vi "checkout.vi"(6 "destroy queue?":bool, 7 "locked by?":string, 8 "error in (no error)":errorcluster) -> (0 "error out":errorcluster, 3 "GenericExperimentController out":refnum<class "GenericExperimentController.lvclass">)   [LabVIEW 2010, in "GenericExperimentController.lvclass"]
uses:
  GenericExperimentController.lvclass
  class_data.vi
  common/classes/GenericComponent/GenericComponent/GenericComponent.lvclass
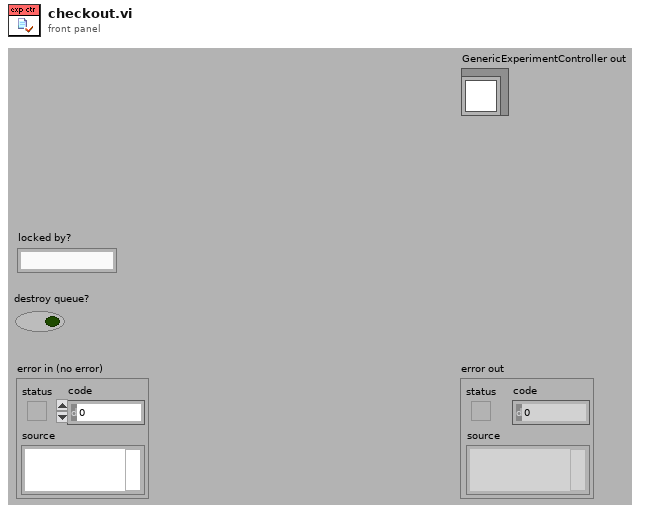
[diagram p1: front panel]
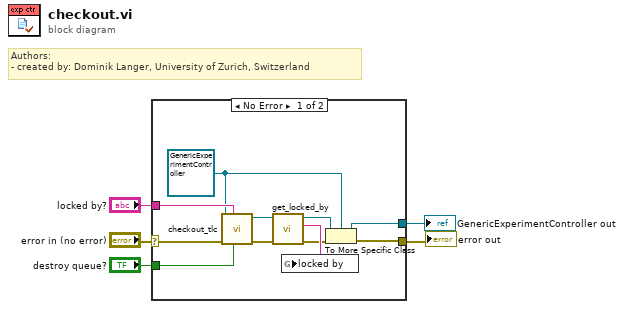
[diagram p0: block diagram]
diagram:
  # "Authors:  \n- created by: Dominik Langer, University of Zurich, Switzerland"
  n1 = case shown="No Error" "error in (no error)" {
    selector: "error in (no error)" -> [w7 w17]
    tunnel: [w15 w17] -> w4
    tunnel: "locked by?" -> [w16 _]
    tunnel: [w14 _] -> w1
    tunnel: "destroy queue?" -> [w8 _]
    frame No Error {
      w6 = refnum<class "GenericExperimentController.lvclass"> refnum ("GenericExperimentController.lvclass")
      n2 = call-dynamic "checkout_tlc.vi"("destroy queue?"=w8, "locked by?"=w16, "error in (no error)"=w7, "GenericToplevelComponent in"=w6) -> ("error out"=w12:errorcluster, "GenericToplevelComponent out"=w11:refnum<class "GenericToplevelComponent.lvclass">)  [unwired: 6 in]
      n3 = call "get_locked_by.vi"("error in (no error)"=w12, "GenericPlugin.lvclass in"=w11) -> ("error out"=w10:errorcluster, "locked by"=w13:string, "GenericPlugin.lvclass out"=w9:refnum<class "GenericToplevelComponent.lvclass">)  [unwired: 7 out]
      n4 = global write "class_data.vi" "locked by"(w13) -> ()
      n5 = To More Specific Class(target class=w6, reference=w9, error in=w10) -> (specific class reference=w14:refnum<class "GenericExperimentController.lvclass">, error out=w15:errorcluster)
    }
    frame Error {
    }
  }
  "error out" <- w4
  "GenericExperimentController out" <- w1
